vi "DAQ Application.vi"() -> ()   [LabVIEW 2025, in "MCP Demo Application.lvlib"]
uses:
  MCP Demo Application.lvlib
  Set Amplitude.vi
  Set Frequency.vi
  Get Waveforms.vi
  Globals.vi
  Joke Creator.vi
  src/MCP Server/MCP Server.lvlib
  <vilib>/JDP Science/JSONtext/JSONtext.lvlib
panel:
  in  "error":bool
  out "value":string
  out "String":string
  in  "Stop":bool
  out "FFT Graph":waveform(dbl)[](graph)
  in  "amplitude\nsweetspot":dbl=6.7
  in  "frequency\nsweetspot":dbl=1.7
  in  "Frequency":dbl(slide) scale=0.0..3.0
  in  "Amplitude":dbl(slide) scale=0.0..14.0
  out "Waveform Chart":waveform(dbl)[](graph)
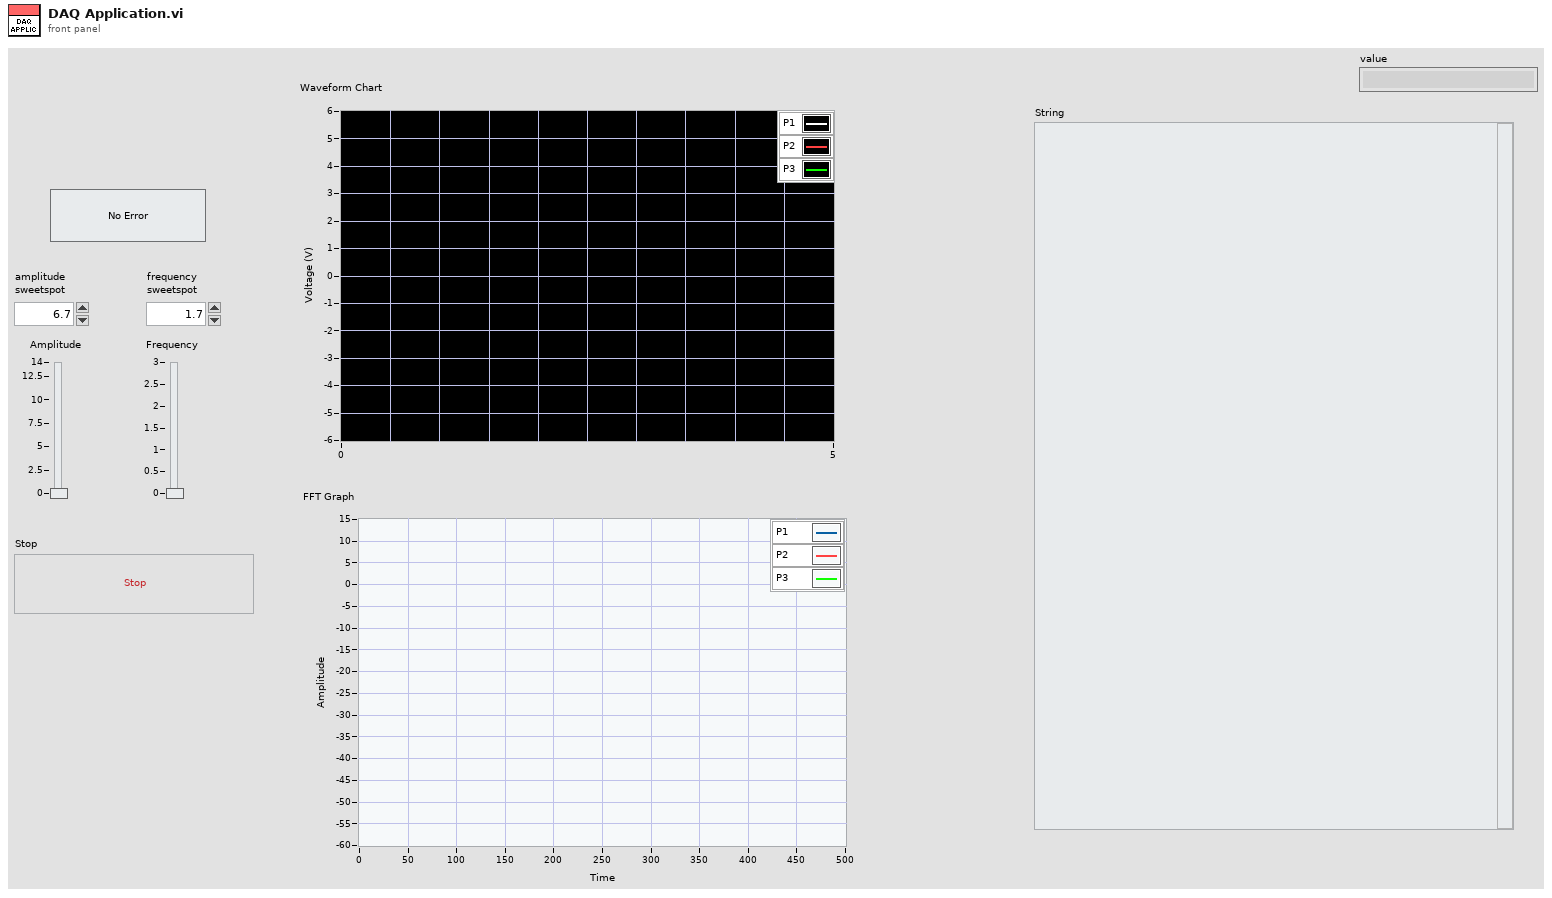
[diagram p1: front panel]
types:
  T1 = typedef "MCP Server.lvlib/User Events.ctl" = cluster{"onError":refnum<user-event>, "onLog":refnum<user-event>, "onConnect":refnum<user-event>, "onToolsList":refnum<user-event>, "onToolsCall":refnum<user-event>, "onNotification":refnum<user-event>, "onTool":refnum<user-event>, "onRpc":refnum<user-event>}
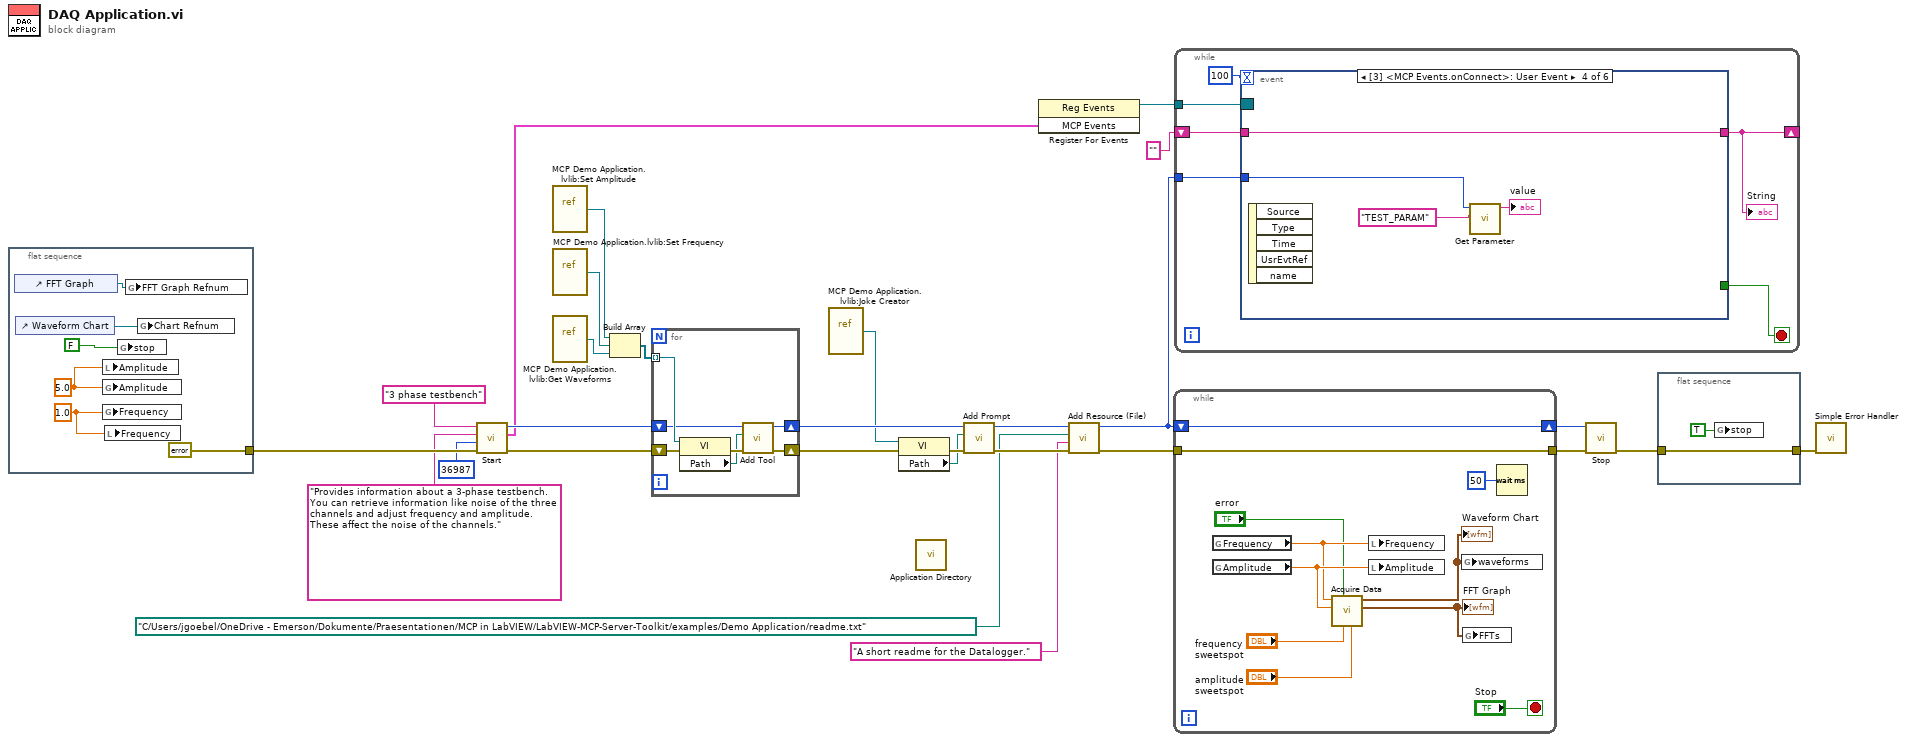
[diagram p0: block diagram]
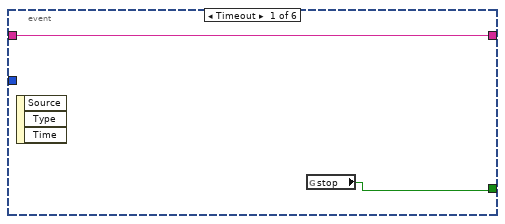
[diagram p2: hidden frame]
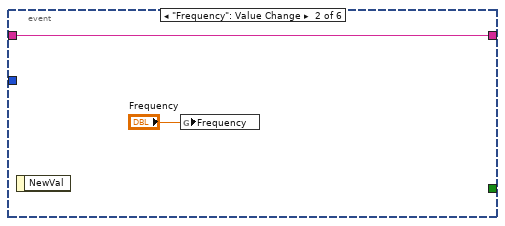
[diagram p3: hidden frame]
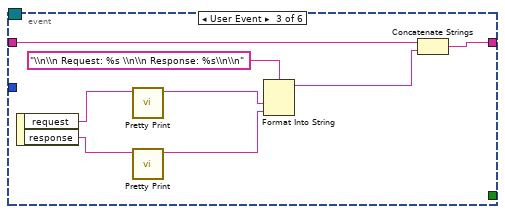
[diagram p4: hidden frame]
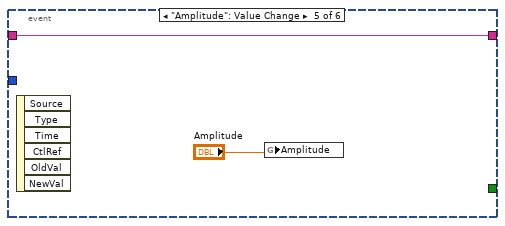
[diagram p5: hidden frame]
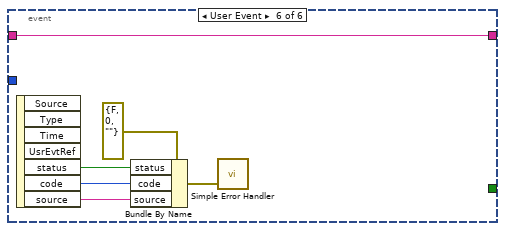
[diagram p6: hidden frame]
diagram:
  n1 = flat-sequence {
    tunnel: [errorcluster {"status"=FALSE, "code"=0, "source"=""} ("error out")] -> w24
    frame #0 {
      w32 = 5.0 ("Amplitude")
      w31 = 1.0 ("Frequency")
      n2 = control-ref of="FFT Graph"() -> (w29:refnum<vi>)
      n3 = control-ref of="Waveform Chart"() -> (w30:refnum<vi>)
      n4 = local write "Amplitude"(w32) -> ()
      n5 = global write "Globals.vi" "Amplitude"(w32) -> ()
      n6 = global write "Globals.vi" "Frequency"(w31) -> ()
      n7 = local write "Frequency"(w31) -> ()
      n8 = global write "Globals.vi" "stop"(FALSE ("stop")) -> ()
      n9 = global write "Globals.vi" "FFT Graph Refnum"(w29) -> ()
      n10 = global write "Globals.vi" "Chart Refnum"(w30) -> ()
    }
  }
  n11 = call "Start.vi"("error in (no error)"=w24, "HTTP Port (36987)"=u16 36987, "Description"="Provides information about a 3-phase testbench. You can retrieve information like noise of the three channels and adjust frequency and amplitude. These affect the noise of the channels." ("Server Description"), "Name"="3 phase testbench" ("Server Name")) -> ("error out"=w21:errorcluster, "MCP Events"=w16:T1, "id out"=w18:i32)  [unwired: 5 in]
  n12 = vi-ref "MCP Demo Application.lvlib:Set Amplitude.vi"() -> (w28:refnum<vi>)
  n13 = vi-ref "MCP Demo Application.lvlib:Set Frequency.vi"() -> (w27:refnum<vi>)
  n14 = vi-ref "MCP Demo Application.lvlib:Get Waveforms.vi"() -> (w26:refnum<vi>)
  n15 = Build Array(w28, w27, w26) -> (w25:refnum<vi>[])
  n16 = for {
    tunnel: w25 -> [w41] mode=indexing
    shift-right: [w40] -> w9
    shift-left: w21 -> [w39]
    shift-right: [w35] -> w11
    shift-left: w18 -> [w36]
    n17 = property class="VI"(reference=w41, error in=w39) -> (error out=w38:errorcluster, "Path"=w37:path)  [unwired: 1 out]
    n18 = call "Add Tool.vi"("error in (no error)"=w38, "vi path"=w37, "id"=w36) -> ("error out"=w40:errorcluster, "id out"=w35:i32)  [unwired: 7 in]
  }
  n19 = vi-ref "MCP Demo Application.lvlib:Joke Creator.vi"() -> (w10:refnum<vi>)
  n20 = property class="VI"(reference=w10, error in=w9) -> (error out=w8:errorcluster, "Path"=w7:path)  [unwired: 1 out]
  n21 = call <vilib>:"Application Directory.vi"() -> ()  [unwired: 1 out]
  n22 = call "Add Prompt.vi"("error in (no error)"=w8, "vi path"=w7, "server id"=w11) -> ("error out"=w12:errorcluster, "server id out"=w5:i32)  [unwired: 7 in]
  n23 = register-events(w16) -> (reference out=w15:refnum<event-registration>)  [unwired: 2 in, 1 out]
  n24 = call "Add Resource (File).vi"("error in (no error)"=w12, "description"="A short readme for the Datalogger.", "file path"=path "C:/Users/jgoebel/OneDrive - Emerson/Dokumente/Praesentationen/MCP in LabVIEW/LabVIEW-MCP-Server-Toolkit/examples/Demo Application/readme.txt", "server id"=w5) -> ("error out"=w6:errorcluster, "server id out"=w4:i32)  [unwired: 6 in]
  n25 = while {
    tunnel: w6 -> [w51]
    tunnel: [w51] -> w23
    shift-right: [w50] -> w17
    shift-left: w4 -> [w50]
    stop <- "Stop" stop-if-true
    n26 = global read "Globals.vi" "Frequency"() -> (w43:dbl)
    n27 = global read "Globals.vi" "Amplitude"() -> (w44:dbl)
    n28 = call "Acquire Data.vi"("amplitude\nsweetspot"="amplitude\nsweetspot", "frequency\nsweetspot"="frequency\nsweetspot", "error"="error", "Amplitude"=w44, "Frequency"=w43) -> ("FFTs"=w48:waveform(dbl)[], "Waveforms"=w47:waveform(dbl)[])  [unwired: 5 in]
    "Waveform Chart" <- w47
    "FFT Graph" <- w48
    n29 = local write "Frequency"(w43) -> ()
    n30 = local write "Amplitude"(w44) -> ()
    n31 = global write "Globals.vi" "waveforms"(w47) -> ()
    n32 = global write "Globals.vi" "FFTs"(w48) -> ()
    n33 = Wait (ms)(milliseconds to wait=u32 50) -> ()  [unwired: 1 out]
  }
  n34 = while {
    tunnel: w15 -> [w58]
    shift-right: [w54] -> _
    shift-left: "" -> [w55]
    tunnel: w4 -> [w53]
    stop <- w57 stop-if-true
    n35 = event shown="[3] <MCP Events.onConnect>: User Event" {
      selector: w58 -> [_ _ _ _ _ _]
      dyn-events: _ -> [_ _ _ _ _ _]
      timeout: 100 -> [_ _ _ _ _ _]
      tunnel: [w60 _ _ _ _ _] -> w57
      tunnel: [w59 w61 w64 w74 w75 w77] -> w54
      tunnel: w55 -> [w59 w61 w65 w74 w75 w77]
      tunnel: w53 -> [_ _ _ w73 _ _]
      event Timeout {
        n36 = event-data() -> ()  [unwired: 1 in, 3 out]
        n37 = global read "Globals.vi" "stop"() -> (w60:bool)
      }
      event "Frequency": Value Change {
        n38 = event-data() -> ()  [unwired: 1 in, 1 out]
        n39 = global write "Globals.vi" "Frequency"("Frequency") -> ()
      }
      event User Event {
        n40 = event-data() -> ("request"=w70:string, "response"=w69:string)  [unwired: 1 in]
        n41 = call <vilib>:"Pretty Print.vi"("JSON"=w70) -> ("<JSON>"=w67:string)  [unwired: 8 in, 2 out]
        n42 = call <vilib>:"Pretty Print.vi"("JSON"=w69) -> ("<JSON>"=w66:string)  [unwired: 8 in, 2 out]
        n43 = Format Into String(format string="\\n\\n Request: %s \\n\\n Response: %s\\n\\n", w67, w66) -> (resulting string=w63:string)  [unwired: 2 in, 1 out]
        n44 = Concatenate Strings(w65, w63) -> (w64:string)
      }
      event User Event {
        n45 = event-data() -> ()  [unwired: 1 in, 5 out]
        n46 = call "Get Parameter.vi"("Name"="TEST_PARAM", "id"=w73) -> ("value"=→"value":string)  [unwired: 7 in, 2 out]
      }
      event "Amplitude": Value Change {
        n47 = event-data() -> ()  [unwired: 1 in, 6 out]
        n48 = global write "Globals.vi" "Amplitude"("Amplitude") -> ()
      }
      event User Event {
        n49 = event-data() -> ("status"=w79:bool, "code"=w80:i32, "source"=w81:string)  [unwired: 1 in, 4 out]
        n50 = Bundle By Name(cluster=errorcluster {"status"=FALSE, "code"=0, "source"=""} ("error constant"), "status"=w79, "code"=w80, "source"=w81) -> (w78:errorcluster)
        n51 = call <vilib>:"Simple Error Handler.vi"("error in (no error)"=w78) -> ()  [unwired: 4 in, 5 out]
      }
    }
    "String" <- w54
  }
  n52 = call "Stop.vi"("error in (no error)"=w23, "id"=w17) -> ("error out"=w22:errorcluster)  [unwired: 9 in]
  n53 = flat-sequence {
    tunnel: w22 -> [w84]
    tunnel: [w84] -> w14
    frame #0 {
      n54 = global write "Globals.vi" "stop"(TRUE ("stop")) -> ()
    }
  }
  n55 = call <vilib>:"Simple Error Handler.vi"("error in (no error)"=w14) -> ()  [unwired: 4 in, 5 out]
